vi "Gauge_Converter_RP.vi"(11 "string":string) -> (3 "decimal":dbl)   [LabVIEW 2014]
uses:
  <vilib>/ptbypt/NI_PtbyPt.lvlib
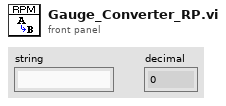
[diagram p1: front panel]
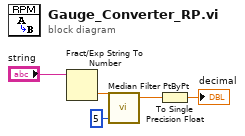
[diagram p0: block diagram]
diagram:
  n1 = Fract/Exp String To Number(string="string") -> (number=w1:dbl)  [unwired: 3 in, 1 out]
  n2 = call <vilib>:"Median Filter PtByPt.vi"("rank"=5, "x"=w1) -> ("Filtered x"=w2:dbl)  [unwired: 2 in, 1 out]
  n3 = To Single Precision Float(number=w2) -> (single precision float=→"decimal":sgl)
